vi "Charts_Graphs_Arrays.vi"() -> ()   [LabVIEW 2015]
panel:
  out "Output \narray":dbl[][](array[numeric])
  out "XY Graph":cluster{"Y":dbl[], "Y":dbl[]}[](graph)
  out "Waveform Graph":dbl[](graph)
  out "Waveform Chart":dbl[](graph)
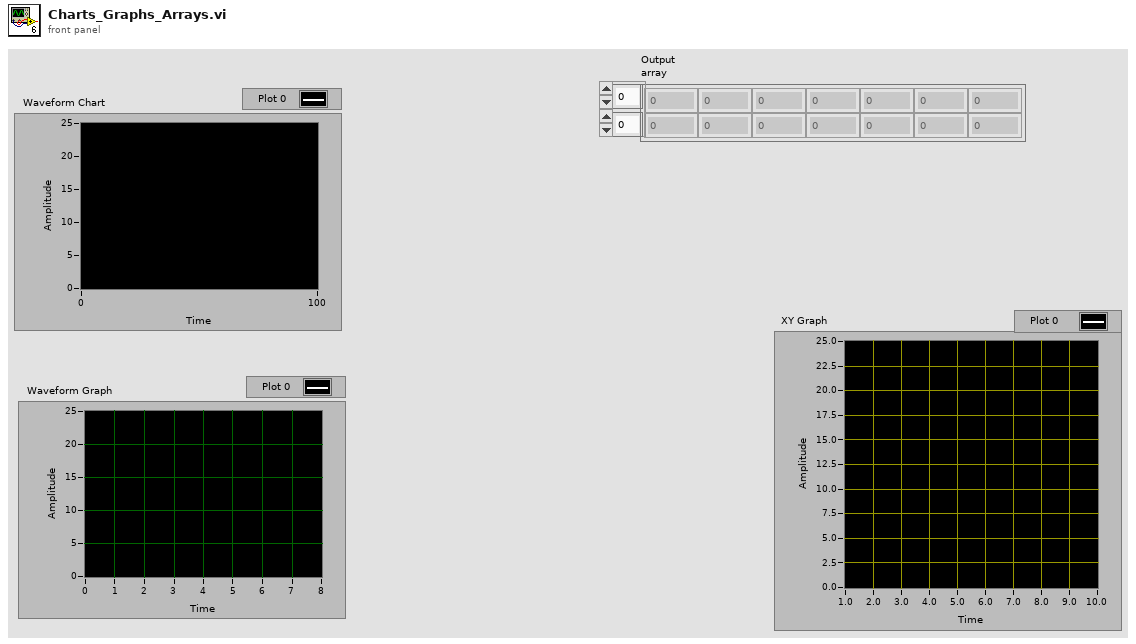
[diagram p1: front panel]
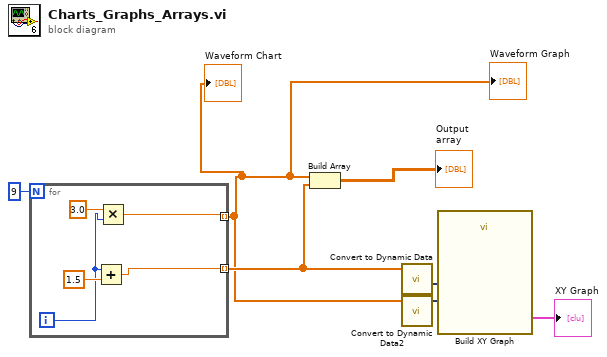
[diagram p0: block diagram]
diagram:
  n1 = for {
    N: 9 -> [_]
    tunnel: [w9] -> w2 mode=indexing
    tunnel: [w8] -> w4 mode=indexing
    i -> [w10]
    n2 = Add(x=w10, y=1.5) -> (x+y=w8:dbl)
    n3 = Multiply(x=3.0, y=w10) -> (x*y=w9:dbl)
  }
  "Waveform Chart" <- w2
  "Waveform Graph" <- w2
  n4 = Build Array(w2, w4) -> (→"Output \narray":dbl[][])
  n5 = call "Convert to Dynamic Data"("Array"=w4) -> ("Dynamic Data Type"=w3:dynamicdata)  [unwired: 3 in]
  n6 = call "Convert to Dynamic Data2"("Array"=w2) -> ("Dynamic Data Type"=w1:dynamicdata)  [unwired: 3 in]
  n7 = call "Build XY Graph"("Y Input"=w1, "X Input"=w3) -> ("XY Graph"=→"XY Graph":cluster{"X":dbl[], "Y":dbl[]}[])  [unwired: 8 in, 1 out]
